vi "Default Instrument Setup.vi"(8 "error in (no error)":errorcluster, 11 "VISA resource name":refnum<visa-resource-name>) -> (0 "error out":errorcluster, 3 "VISA resource name out":refnum<visa-resource-name>)   [LabVIEW 2012, in "Keysight B2980 Series.lvlib"]
doc: "Sends a default command string to the instrument whenever a new VISA session is opened, or the instrument is reset. Use this VI as a subVI for the Initialize and Reset VIs. Altering this VI could cause these two VIs to operate incorrectly."
uses:
  Keysight B2980 Series.lvlib
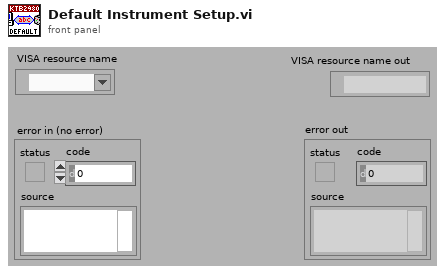
[diagram p1: front panel]
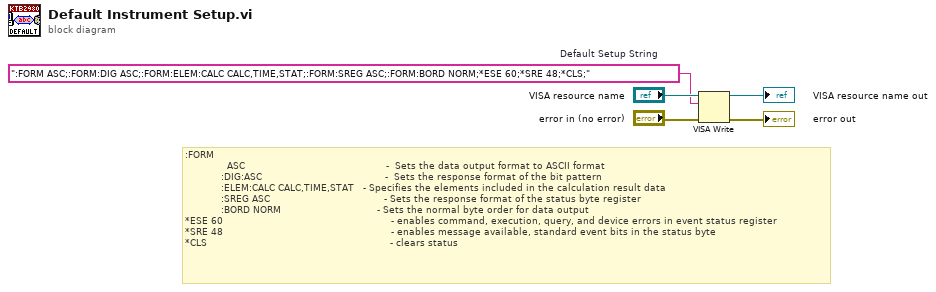
[diagram p0: block diagram]
diagram:
  w1 = ":FORM ASC;:FORM:DIG ASC;:FORM:ELEM:CALC CALC,TIME,STAT;:FORM:SREG ASC;:FORM:BORD NORM;*ESE 60;*SRE 48;*CLS;"  # Default Setup String
  # ":FORM\n              ASC                                               -  Sets the data output format to ASCII format\n            :DIG:ASC                                         -  Sets the response format of the bit pattern \n            :ELEM:CALC CALC,TIME,STAT   - Specifies the elements included in the calculation result data \n            :SREG ASC                                      - Sets the response format of the status byte register\n            :BORD NORM                                - Sets the normal byte order for data output\n*ESE 60                                                        - enables command, execution, query, and device errors in event status register\n*SRE 48                                                        - enables message available, standard event bits in the status byte\n*CLS                                                             - clears status"
  n1 = VISA Write(VISA resource name="VISA resource name", write buffer=w1, error in (no error)="error in (no error)") -> (VISA resource name out=→"VISA resource name out":refnum<visa-resource-name>, error out=→"error out":errorcluster)  [unwired: 1 out]
